vi "xml_get_use.vi"(0 "target name":string, 1 "XML Path":path=path "D:/Test Management/Farmer/XML/targets.xml", 2 "error in (no error)":errorcluster) -> (3 "in use?":bool, 4 "user":string, 5 "success?":bool, 6 "error out":errorcluster)   [LabVIEW 2011]
uses:
  <vilib>/xml/Load XML File.vi
  <vilib>/xml/Close Reference(Node).vi
  <vilib>/xml/NI_XML.lvlib
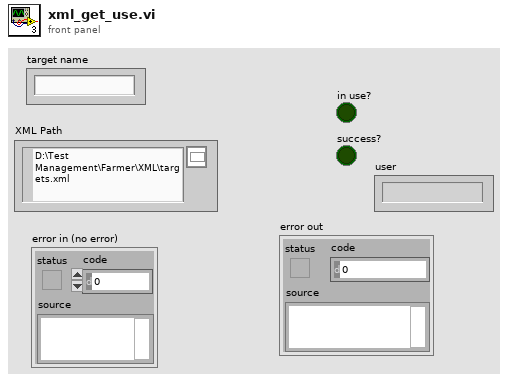
[diagram p1: front panel]
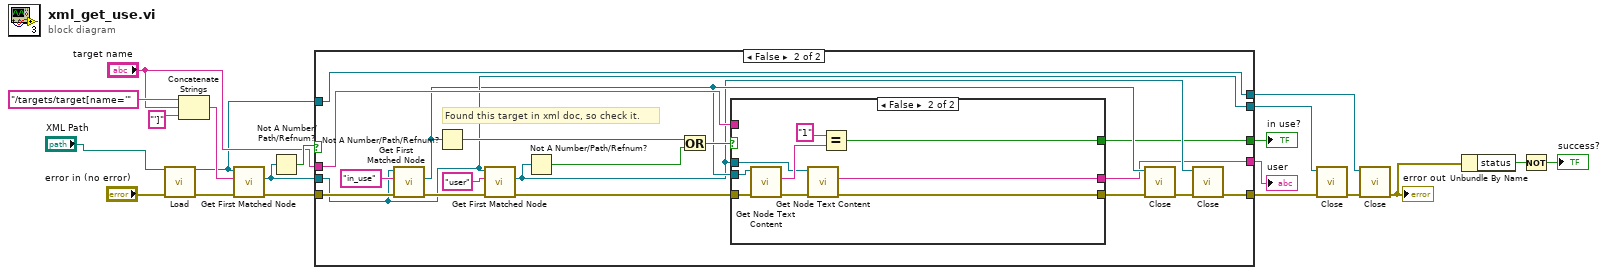
[diagram p0: block diagram]
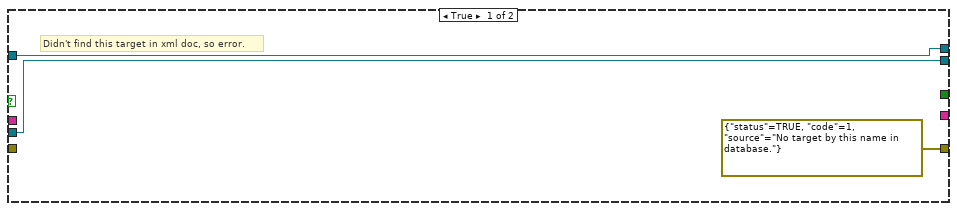
[diagram p2: hidden frame]
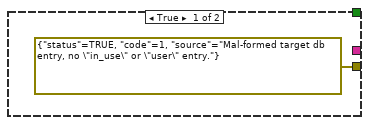
[diagram p3: hidden frame]
diagram:
  n1 = call-poly <vilib>:"Load.vi"("path to XML document"="XML Path", "error in (no error)"="error in (no error)") -> ("DOM document out"=w5:refnum<k20>, "error out"=w17:errorcluster)  [unwired: 11 in, 1 out]
  n2 = Concatenate Strings("/targets/target[name='", "target name", "']") -> (w18:string)
  n3 = call <vilib>:"Get First Matched Node.vi"("error in (no error)"=w17, "XPath expression"=w18, "node in"=w5) -> ("error out"=w16:errorcluster, "node result"=w13:refnum<k20>)  [unwired: 6 in, 1 out]
  n4 = Not A Number/Path/Refnum?(number/path/refnum=w13) -> (NaN/Path/Refnum?=w15:bool)
  n5 = case shown="False" w15 {
    tunnel: w16 -> [_ w41]
    tunnel: [errorcluster {"status"=TRUE, "code"=1, "source"="No target by this name in database."} ("error out") w28] -> w7
    tunnel: w13 -> [w22 w32]
    tunnel: "target name" -> [_ w33]
    tunnel: [w22 w32] -> w6
    tunnel: w5 -> [w21 w31]
    tunnel: [w21 w31] -> w4
    tunnel: [_ w25] -> w3
    tunnel: [_ w24] -> w2
    frame True {
      # "Didn't find this target in xml doc, so error."
    }
    frame False {
      # "Found this target in xml doc, so check it."
      n6 = call <vilib>:"Get First Matched Node.vi"("error in (no error)"=w41, "XPath expression"="in_use", "node in"=w32) -> ("error out"=w36:errorcluster, "node result"=w27:refnum<k20>)  [unwired: 6 in, 1 out]
      n7 = Not A Number/Path/Refnum?(number/path/refnum=w27) -> (NaN/Path/Refnum?=w39:bool)
      n8 = call <vilib>:"Get First Matched Node.vi"("error in (no error)"=w36, "XPath expression"="user", "node in"=w32) -> ("error out"=w35:errorcluster, "node result"=w26:refnum<k20>)  [unwired: 6 in, 1 out]
      n9 = Not A Number/Path/Refnum?(number/path/refnum=w26) -> (NaN/Path/Refnum?=w37:bool)
      n10 = Or(x=w39, y=w37) -> (x .or. y?=w38:bool)
      n11 = case shown="False" w38 {
        tunnel: [errorcluster {"status"=TRUE, "code"=1, "source"="Mal-formed target db entry, no \"in_use\" or \"user\" entry."} ("error out") w45] -> w29
        tunnel: w27 -> [_ w51]
        tunnel: w35 -> [_ w50]
        tunnel: w26 -> [_ w48]
        tunnel: w33 -> [_ _]
        tunnel: [_ w44] -> w25
        tunnel: [_ w43] -> w24
        frame True {
        }
        frame False {
          n12 = call <vilib>:"Get Node Text Content.vi"("error in (no error)"=w50, "node in"=w51) -> ("error out"=w47:errorcluster, "node text"=w49:string)  [unwired: 7 in, 1 out]
          n13 = call <vilib>:"Get Node Text Content.vi"("error in (no error)"=w47, "node in"=w48) -> ("error out"=w45:errorcluster, "node text"=w43:string)  [unwired: 7 in, 1 out]
          n14 = Equal?(x="1", y=w49) -> (x = y?=w44:bool)
        }
      }
      n15 = call-poly <vilib>:"Close.vi"("error in (no error)"=w29, "node"=w27) -> ("error out"=w30:errorcluster)  [unwired: 7 in]
      n16 = call-poly <vilib>:"Close.vi"("error in (no error)"=w30, "node"=w26) -> ("error out"=w28:errorcluster)  [unwired: 7 in]
    }
  }
  "in use?" <- w3
  "user" <- w2
  n17 = call-poly <vilib>:"Close.vi"("error in (no error)"=w7, "node"=w6) -> ("error out"=w14:errorcluster)  [unwired: 7 in]
  n18 = call-poly <vilib>:"Close.vi"("error in (no error)"=w14, "node"=w4) -> ("error out"=w11:errorcluster)  [unwired: 7 in]
  "error out" <- w11
  n19 = Unbundle By Name(w11) -> ("status"=w10:bool)
  n20 = Not(x=w10) -> (.not. x?=→"success?":bool)
